vi "TC1014.vi"() -> ()   [LabVIEW 2019]
uses:
  SubVI/Typedef/TLibCANFD.ctl
panel:
  in  "启用4通道":bool
  in  "启用3通道":bool
  in  "启用2通道":bool
  in  "启用1通道":bool
  in  "选项卡控件":enum32{"CANFD1", "CANFD2", "CANFD3", "CANFD4"}(tab)
  in  "CH1  FD帧":u8(ring) items=["普通 CAN数据", "FD CAN数据"]
  in  "CH1显示报文类型":u16(ring)=1 items=["只读取接收的报文", "接收报文&发送报文"]
  in  "CH1终端电阻":u16(ring)=1 items=["Disable", "Enable"]
  in  "CH1物理通道":i32(ring) items=["CHN1", "CHN2", "CHN3", "CHN4", "CHN5", "CHN6", "CHN7", "CHN8", "CHN9", "CHN10", "CHN11", "CHN12", "CHN13", "CHN14", "CHN15", "CHN16", "CHN17", "CHN18", "CHN19", "CHN20", "CHN21", "CHN22", "CHN23", "CHN24", "CHN25", "CHN26", "CHN27", "CHN28", "CHN29", "CHN30", "CHN31", "CHN32"]
  in  "CH1应用程序逻辑通道":i32(ring) items=["CHN1", "CHN2", "CHN3", "CHN4", "CHN5", "CHN6", "CHN7", "CHN8", "CHN9", "CHN10", "CHN11", "CHN12", "CHN13", "CHN14", "CHN15", "CHN16", "CHN17", "CHN18", "CHN19", "CHN20", "CHN21", "CHN22", "CHN23", "CHN24", "CHN25", "CHN26", "CHN27", "CHN28", "CHN29", "CHN30", "CHN31", "CHN32"]
  in  "CH1仲裁域波特率":sgl=500.0 format="%#_g k"
  in  "CH1数据域波特率":sgl=2000.0 format="%#_g k"
  in  "CH1控制器类型":i32(ring)=1 items=["lfdtCAN", "lfdtISOFDCAN", "lfdtNonISOFDFDCAN"]
  in  "CH1控制器工作模式":i32(ring) items=["lfdmNormal", "lfdmACKOff", "lfdmRestricted"]
  in  "CH1发送":bool
  in  "CH1ID":i32 format="%x"
  in  "CH1帧格式":u8(ring) items=["标准帧", "扩展帧"]
  in  "CH1帧类型":u8(ring) items=["数据帧", "远程帧"]
  in  "CH1长度":u8
  in  "CH1SendData":u8[](array[numeric])=[0, 0, 0, 0, 0, 0, 0, 0, 0, 0, 0, 0, 0, 0, 0, 0, 0, 0, 0, 0, 0, 0, 0, 0, 0, 0, 0, 0, 0, 0, 0, 0, 0, 0, 0, 0, 0, 0, 0, 0, 0, 0, 0, 0, 0, 0, 0, 0, 0, 0, 0, 0, 0, 0, 0, 0, 0, 0, 0, 0, 0, 0, 0, 0, 0, 0, 0, 0, 0, 0, 0, 0, 0, 0, 0, 0] format="%x"
  in  "CH1Data":i32(listbox)=-1
  in  "CH2 FD帧 2":u8(ring) items=["普通 CAN数据", "FD CAN数据"]
  in  "CH2显示报文类型":u16(ring)=1 items=["Rx", "Rx&Tx"]
  in  "CH2终端电阻":u16(ring)=1 items=["Disable", "Enable"]
  in  "CH2物理通道":i32(ring)=1 items=["CHN1", "CHN2", "CHN3", "CHN4", "CHN5", "CHN6", "CHN7", "CHN8", "CHN9", "CHN10", "CHN11", "CHN12", "CHN13", "CHN14", "CHN15", "CHN16", "CHN17", "CHN18", "CHN19", "CHN20", "CHN21", "CHN22", "CHN23", "CHN24", "CHN25", "CHN26", "CHN27", "CHN28", "CHN29", "CHN30", "CHN31", "CHN32"]
  in  "CH2虚拟通道":i32(ring)=1 items=["CHN1", "CHN2", "CHN3", "CHN4", "CHN5", "CHN6", "CHN7", "CHN8", "CHN9", "CHN10", "CHN11", "CHN12", "CHN13", "CHN14", "CHN15", "CHN16", "CHN17", "CHN18", "CHN19", "CHN20", "CHN21", "CHN22", "CHN23", "CHN24", "CHN25", "CHN26", "CHN27", "CHN28", "CHN29", "CHN30", "CHN31", "CHN32"]
  in  "CH2仲裁域波特率":sgl=500.0 format="%#_g k"
  in  "CH2数据域波特率":sgl=2000.0 format="%#_g k"
  in  "CH2控制器类型":i32(ring) items=["lfdtCAN", "lfdtISOFDCAN", "lfdtNonISOFDFDCAN"]
  in  "CH2控制器工作模式":i32(ring) items=["lfdmNormal", "lfdmACKOff", "lfdmRestricted"]
  in  "CH2发送":bool
  in  "CH2ID":i32 format="%x"
  in  "CH2帧格式":u8(ring) items=["标准帧", "扩展帧"]
  in  "CH2帧类型":u8(ring) items=["数据帧", "远程帧"]
  in  "CH2长度":u8
  in  "CH2SendData":u8[](array[numeric])=[0, 0, 0, 0, 0, 0, 0, 0, 0, 0, 0, 0, 0, 0, 0, 0, 0, 0, 0, 0, 0, 0, 0, 0, 0, 0, 0, 0, 0, 0, 0, 0, 0, 0, 0, 0, 0, 0, 0, 0, 0, 0, 0, 0, 0, 0, 0, 0, 0, 0, 0, 0, 0, 0, 0, 0, 0, 0, 0, 0, 0, 0, 0, 0, 0, 0, 0, 0, 0, 0, 0, 0, 0, 0, 0, 0] format="%x"
  in  "CH2Data":i32(listbox)=-1
  in  "CH3 FD帧 3":u8(ring) items=["普通 CAN数据", "FD CAN数据"]
  in  "CH3显示报文类型":u16(ring)=1 items=["Rx", "Rx&Tx"]
  in  "CH3终端电阻":u16(ring)=1 items=["Disable", "Enable"]
  in  "CH3物理通道":i32(ring)=2 items=["CHN1", "CHN2", "CHN3", "CHN4", "CHN5", "CHN6", "CHN7", "CHN8", "CHN9", "CHN10", "CHN11", "CHN12", "CHN13", "CHN14", "CHN15", "CHN16", "CHN17", "CHN18", "CHN19", "CHN20", "CHN21", "CHN22", "CHN23", "CHN24", "CHN25", "CHN26", "CHN27", "CHN28", "CHN29", "CHN30", "CHN31", "CHN32"]
  in  "CH3虚拟通道":i32(ring)=2 items=["CHN1", "CHN2", "CHN3", "CHN4", "CHN5", "CHN6", "CHN7", "CHN8", "CHN9", "CHN10", "CHN11", "CHN12", "CHN13", "CHN14", "CHN15", "CHN16", "CHN17", "CHN18", "CHN19", "CHN20", "CHN21", "CHN22", "CHN23", "CHN24", "CHN25", "CHN26", "CHN27", "CHN28", "CHN29", "CHN30", "CHN31", "CHN32"]
  in  "CH3仲裁域波特率":sgl=500.0 format="%#_g k"
  in  "CH3数据域波特率":sgl=2000.0 format="%#_g k"
  in  "CH3控制器类型":i32(ring)=1 items=["lfdtCAN", "lfdtISOFDCAN", "lfdtNonISOFDFDCAN"]
  in  "CH3控制器工作模式":i32(ring) items=["lfdmNormal", "lfdmACKOff", "lfdmRestricted"]
  in  "CH3发送":bool
  in  "CH3ID":i32 format="%x"
  in  "CH3帧格式":u8(ring) items=["标准帧", "扩展帧"]
  in  "CH3帧类型":u8(ring) items=["数据帧", "远程帧"]
  in  "CH3长度":u8
  in  "CH3SendData":u8[](array[numeric])=[0, 0, 0, 0, 0, 0, 0, 0, 0, 0, 0, 0, 0, 0, 0, 0, 0, 0, 0, 0, 0, 0, 0, 0, 0, 0, 0, 0, 0, 0, 0, 0, 0, 0, 0, 0, 0, 0, 0, 0, 0, 0, 0, 0, 0, 0, 0, 0, 0, 0, 0, 0, 0, 0, 0, 0, 0, 0, 0, 0, 0, 0, 0, 0, 0, 0, 0, 0, 0, 0, 0, 0, 0, 0, 0, 0] format="%x"
  in  "CH3Data":i32(listbox)=-1
  in  "CH4 FD帧 3":u8(ring) items=["普通 CAN数据", "FD CAN数据"]
  in  "CH4显示报文类型":u16(ring)=1 items=["Rx", "Rx&Tx"]
  in  "CH4终端电阻":u16(ring)=1 items=["Disable", "Enable"]
  in  "CH4物理通道":i32(ring)=3 items=["CHN1", "CHN2", "CHN3", "CHN4", "CHN5", "CHN6", "CHN7", "CHN8", "CHN9", "CHN10", "CHN11", "CHN12", "CHN13", "CHN14", "CHN15", "CHN16", "CHN17", "CHN18", "CHN19", "CHN20", "CHN21", "CHN22", "CHN23", "CHN24", "CHN25", "CHN26", "CHN27", "CHN28", "CHN29", "CHN30", "CHN31", "CHN32"]
  in  "CH4虚拟通道":i32(ring)=3 items=["CHN1", "CHN2", "CHN3", "CHN4", "CHN5", "CHN6", "CHN7", "CHN8", "CHN9", "CHN10", "CHN11", "CHN12", "CHN13", "CHN14", "CHN15", "CHN16", "CHN17", "CHN18", "CHN19", "CHN20", "CHN21", "CHN22", "CHN23", "CHN24", "CHN25", "CHN26", "CHN27", "CHN28", "CHN29", "CHN30", "CHN31", "CHN32"]
  in  "CH4仲裁域波特率":sgl=500.0 format="%#_g k"
  in  "CH4数据域波特率":sgl=2000.0 format="%#_g k"
  in  "CH4控制器类型":i32(ring)=1 items=["lfdtCAN", "lfdtISOFDCAN", "lfdtNonISOFDFDCAN"]
  in  "CH4控制器工作模式":i32(ring) items=["lfdmNormal", "lfdmACKOff", "lfdmRestricted"]
  in  "CH4发送":bool
  in  "CH4ID":i32 format="%x"
  in  "CH4帧格式":u8(ring) items=["标准帧", "扩展帧"]
  in  "CH4帧类型":u8(ring) items=["数据帧", "远程帧"]
  in  "CH4长度":u8
  in  "CH4SendData":u8[](array[numeric])=[0, 0, 0, 0, 0, 0, 0, 0, 0, 0, 0, 0, 0, 0, 0, 0, 0, 0, 0, 0, 0, 0, 0, 0, 0, 0, 0, 0, 0, 0, 0, 0, 0, 0, 0, 0, 0, 0, 0, 0, 0, 0, 0, 0, 0, 0, 0, 0, 0, 0, 0, 0, 0, 0, 0, 0, 0, 0, 0, 0, 0, 0, 0, 0, 0, 0, 0, 0, 0, 0, 0, 0, 0, 0, 0, 0] format="%x"
  in  "CH4Data":i32(listbox)=-1
  out "通讯":bool
  in  "使用通道数量":u16(ring)=4 items=["1通道"=1, "2通道"=2, "3通道"=3, "4通道"=4, "5通道"=5]
  in  "硬件启闭":bool
  in  "退出程序":bool
  # "CAN DEMO_TC1014"
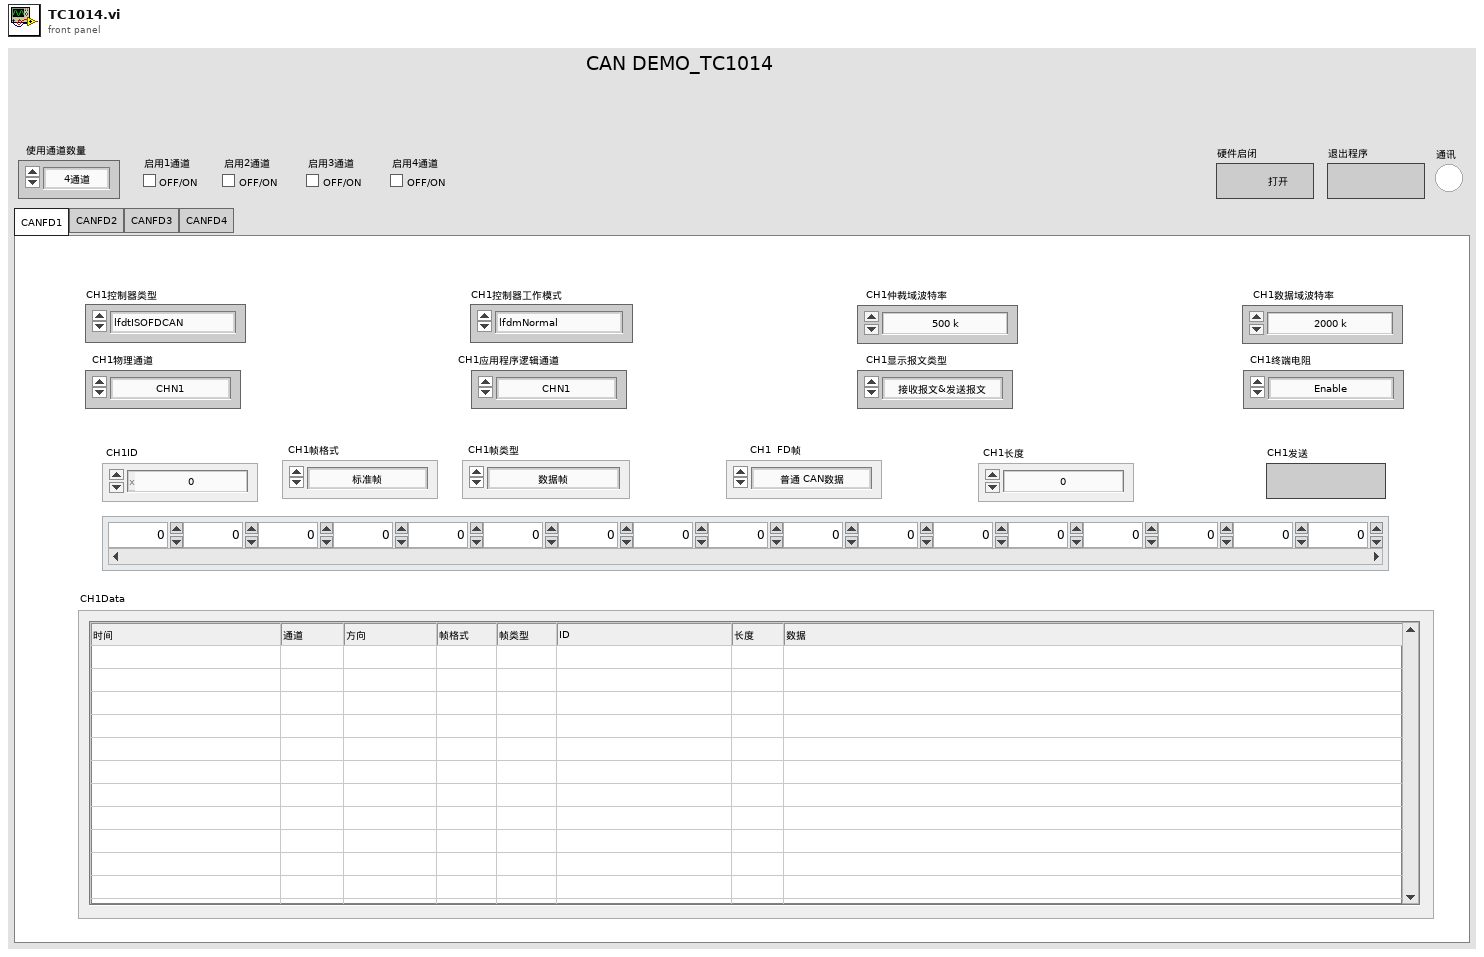
[diagram p1: front panel]
types:
  T1 = cluster{"AIdxchn":u8, "AId":i32, "AIsStd":u8, "AIsData":u8, "ADLC":u8, "簇":cluster{"初始化的数组[0]":u8, "初始化的数组[1]":u8, "初始化的数组[2]":u8, "初始化的数组[3]":u8, "初始化的数组[4]":u8, "初始化的数组[5]":u8, "初始化的数组[6]":u8, "初始化的数组[7]":u8, "初始化的数组[8]":u8, "初始化的数组[9]":u8, "初始化的数组[10]":u8, "初始化的数组[11]":u8, "初始化的数组[12]":u8, "初始化的数组[13]":u8, "初始化的数组[14]":u8, "初始化的数组[15]":u8, "初始化的数组[16]":u8, "初始化的数组[17]":u8, "初始化的数组[18]":u8, "初始化的数组[19]":u8, "初始化的数组[20]":u8, "初始化的数组[21]":u8, "初始化的数组[22]":u8, "初始化的数组[23]":u8, "初始化的数组[24]":u8, "初始化的数组[25]":u8, "初始化的数组[26]":u8, "初始化的数组[27]":u8, "初始化的数组[28]":u8, "初始化的数组[29]":u8, "初始化的数组[30]":u8, "初始化的数组[31]":u8, "初始化的数组[32]":u8, "初始化的数组[33]":u8, "初始化的数组[34]":u8, "初始化的数组[35]":u8, "初始化的数组[36]":u8, "初始化的数组[37]":u8, "初始化的数组[38]":u8, "初始化的数组[39]":u8, "初始化的数组[40]":u8, "初始化的数组[41]":u8, "初始化的数组[42]":u8, "初始化的数组[43]":u8, "初始化的数组[44]":u8, "初始化的数组[45]":u8, "初始化的数组[46]":u8, "初始化的数组[47]":u8, "初始化的数组[48]":u8, "初始化的数组[49]":u8, "初始化的数组[50]":u8, "初始化的数组[51]":u8, "初始化的数组[52]":u8, "初始化的数组[53]":u8, "初始化的数组[54]":u8, "初始化的数组[55]":u8, "初始化的数组[56]":u8, "初始化的数组[57]":u8, "初始化的数组[58]":u8, "初始化的数组[59]":u8, "初始化的数组[60]":u8, "初始化的数组[61]":u8, "初始化的数组[62]":u8, "初始化的数组[63]":u8, "初始化的数组[64] ":u8}}
  T2 = cluster{"FIdxChn":u8, "FProperties":u8, "FDLC":u8, "FReserved":u8, "FIdentifier":i32, "FTimeUS":u64, "簇":cluster{"初始化的数组[0]":u8, "初始化的数组[1]":u8, "初始化的数组[2]":u8, "初始化的数组[3]":u8, "初始化的数组[4]":u8, "初始化的数组[5]":u8, "初始化的数组[6]":u8, "初始化的数组[7]":u8, "初始化的数组[8]":u8, "初始化的数组[9]":u8, "初始化的数组[10]":u8, "初始化的数组[11]":u8, "初始化的数组[12]":u8, "初始化的数组[13]":u8, "初始化的数组[14]":u8, "初始化的数组[15]":u8, "初始化的数组[16]":u8, "初始化的数组[17]":u8, "初始化的数组[18]":u8, "初始化的数组[19]":u8, "初始化的数组[20]":u8, "初始化的数组[21]":u8, "初始化的数组[22]":u8, "初始化的数组[23]":u8, "初始化的数组[24]":u8, "初始化的数组[25]":u8, "初始化的数组[26]":u8, "初始化的数组[27]":u8, "初始化的数组[28]":u8, "初始化的数组[29]":u8, "初始化的数组[30]":u8, "初始化的数组[31]":u8, "初始化的数组[32]":u8, "初始化的数组[33]":u8, "初始化的数组[34]":u8, "初始化的数组[35]":u8, "初始化的数组[36]":u8, "初始化的数组[37]":u8, "初始化的数组[38]":u8, "初始化的数组[39]":u8, "初始化的数组[40]":u8, "初始化的数组[41]":u8, "初始化的数组[42]":u8, "初始化的数组[43]":u8, "初始化的数组[44]":u8, "初始化的数组[45]":u8, "初始化的数组[46]":u8, "初始化的数组[47]":u8, "初始化的数组[48]":u8, "初始化的数组[49]":u8, "初始化的数组[50]":u8, "初始化的数组[51]":u8, "初始化的数组[52]":u8, "初始化的数组[53]":u8, "初始化的数组[54]":u8, "初始化的数组[55]":u8, "初始化的数组[56]":u8, "初始化的数组[57]":u8, "初始化的数组[58]":u8, "初始化的数组[59]":u8, "初始化的数组[60]":u8, "初始化的数组[61]":u8, "初始化的数组[62]":u8, "初始化的数组[63]":u8}}[]
  T3 = cluster{"硬件类型":i32, "硬件子类型":i32, "AArbRateKbps":sgl, "AListenOnly":enum16{"Normal", "ListenOnly"}, "Int120Ohm":enum16{"Disable", "Enable"}, "EnableChannel":enum16{"Disable", "Enable"}, "AHwChannel":i32, "AAppChannel":i32, "ADataRateKbps":sgl, "AControllerType":i32, "AControllerMode":i32}
  T4 = typedef "TLibCANFD.ctl" = cluster{"AIdxchn":u8, "AId":i32, "AIsStd":u8, "AIsData":u8, "ADLC":u8, "AIsFD":enum16{"Classic CAN报文", "FD CAN报文"}, "FDatas":cluster{"初始化的数组[0]":u8, "初始化的数组[1]":u8, "初始化的数组[2]":u8, "初始化的数组[3]":u8, "初始化的数组[4]":u8, "初始化的数组[5]":u8, "初始化的数组[6]":u8, "初始化的数组[7]":u8, "初始化的数组[8]":u8, "初始化的数组[9]":u8, "初始化的数组[10]":u8, "初始化的数组[11]":u8, "初始化的数组[12]":u8, "初始化的数组[13]":u8, "初始化的数组[14]":u8, "初始化的数组[15]":u8, "初始化的数组[16]":u8, "初始化的数组[17]":u8, "初始化的数组[18]":u8, "初始化的数组[19]":u8, "初始化的数组[20]":u8, "初始化的数组[21]":u8, "初始化的数组[22]":u8, "初始化的数组[23]":u8, "初始化的数组[24]":u8, "初始化的数组[25]":u8, "初始化的数组[26]":u8, "初始化的数组[27]":u8, "初始化的数组[28]":u8, "初始化的数组[29]":u8, "初始化的数组[30]":u8, "初始化的数组[31]":u8, "初始化的数组[32]":u8, "初始化的数组[33]":u8, "初始化的数组[34]":u8, "初始化的数组[35]":u8, "初始化的数组[36]":u8, "初始化的数组[37]":u8, "初始化的数组[38]":u8, "初始化的数组[39]":u8, "初始化的数组[40]":u8, "初始化的数组[41]":u8, "初始化的数组[42]":u8, "初始化的数组[43]":u8, "初始化的数组[44]":u8, "初始化的数组[45]":u8, "初始化的数组[46]":u8, "初始化的数组[47]":u8, "初始化的数组[48]":u8, "初始化的数组[49]":u8, "初始化的数组[50]":u8, "初始化的数组[51]":u8, "初始化的数组[52]":u8, "初始化的数组[53]":u8, "初始化的数组[54]":u8, "初始化的数组[55]":u8, "初始化的数组[56]":u8, "初始化的数组[57]":u8, "初始化的数组[58]":u8, "初始化的数组[59]":u8, "初始化的数组[60]":u8, "初始化的数组[61]":u8, "初始化的数组[62]":u8, "初始化的数组[63]":u8, "初始化的数组[64] ":u8}}
  T5 = cluster{"CH1SendData[0]":u8, "CH1SendData[1]":u8, "CH1SendData[2]":u8, "CH1SendData[3]":u8, "CH1SendData[4]":u8, "CH1SendData[5]":u8, "CH1SendData[6]":u8, "CH1SendData[7]":u8, "CH1SendData[8]":u8, "CH1SendData[9]":u8, "CH1SendData[10]":u8, "CH1SendData[11]":u8, "CH1SendData[12]":u8, "CH1SendData[13]":u8, "CH1SendData[14]":u8, "CH1SendData[15]":u8, "CH1SendData[16]":u8, "CH1SendData[17]":u8, "CH1SendData[18]":u8, "CH1SendData[19]":u8, "CH1SendData[20]":u8, "CH1SendData[21]":u8, "CH1SendData[22]":u8, "CH1SendData[23]":u8, "CH1SendData[24]":u8, "CH1SendData[25]":u8, "CH1SendData[26]":u8, "CH1SendData[27]":u8, "CH1SendData[28]":u8, "CH1SendData[29]":u8, "CH1SendData[30]":u8, "CH1SendData[31]":u8, "CH1SendData[32]":u8, "CH1SendData[33]":u8, "CH1SendData[34]":u8, "CH1SendData[35]":u8, "CH1SendData[36]":u8, "CH1SendData[37]":u8, "CH1SendData[38]":u8, "CH1SendData[39]":u8, "CH1SendData[40]":u8, "CH1SendData[41]":u8, "CH1SendData[42]":u8, "CH1SendData[43]":u8, "CH1SendData[44]":u8, "CH1SendData[45]":u8, "CH1SendData[46]":u8, "CH1SendData[47]":u8, "CH1SendData[48]":u8, "CH1SendData[49]":u8, "CH1SendData[50]":u8, "CH1SendData[51]":u8, "CH1SendData[52]":u8, "CH1SendData[53]":u8, "CH1SendData[54]":u8, "CH1SendData[55]":u8, "CH1SendData[56]":u8, "CH1SendData[57]":u8, "CH1SendData[58]":u8, "CH1SendData[59]":u8, "CH1SendData[60]":u8, "CH1SendData[61]":u8, "CH1SendData[62]":u8, "CH1SendData[63]":u8, "CH1SendData[64]":u8}
  T6 = cluster{"FIdxChn":u8, "FProperties":u8, "FDLC":u8, "FReserved":u8, "FIdentifier":i32, "FTimeUS":u64, "FData":cluster{"Data0":u8, "Data1":u8, "Data2":u8, "Data3":u8, "Data4":u8, "Data5":u8, "Data6":u8, "Data7":u8}}[]
  T7 = cluster{"FIdxChn":u8, "FProperties":u8, "FDLC":u8, "FReserved":u8, "FIdentifier":i32, "FTimeUS":u64, "Fdata":cluster{"初始化的数组[0]":u8, "初始化的数组[1]":u8, "初始化的数组[2]":u8, "初始化的数组[3]":u8, "初始化的数组[4]":u8, "初始化的数组[5]":u8, "初始化的数组[6]":u8, "初始化的数组[7]":u8, "初始化的数组[8]":u8, "初始化的数组[9]":u8, "初始化的数组[10]":u8, "初始化的数组[11]":u8, "初始化的数组[12]":u8, "初始化的数组[13]":u8, "初始化的数组[14]":u8, "初始化的数组[15]":u8, "初始化的数组[16]":u8, "初始化的数组[17]":u8, "初始化的数组[18]":u8, "初始化的数组[19]":u8, "初始化的数组[20]":u8, "初始化的数组[21]":u8, "初始化的数组[22]":u8, "初始化的数组[23]":u8, "初始化的数组[24]":u8, "初始化的数组[25]":u8, "初始化的数组[26]":u8, "初始化的数组[27]":u8, "初始化的数组[28]":u8, "初始化的数组[29]":u8, "初始化的数组[30]":u8, "初始化的数组[31]":u8, "初始化的数组[32]":u8, "初始化的数组[33]":u8, "初始化的数组[34]":u8, "初始化的数组[35]":u8, "初始化的数组[36]":u8, "初始化的数组[37]":u8, "初始化的数组[38]":u8, "初始化的数组[39]":u8, "初始化的数组[40]":u8, "初始化的数组[41]":u8, "初始化的数组[42]":u8, "初始化的数组[43]":u8, "初始化的数组[44]":u8, "初始化的数组[45]":u8, "初始化的数组[46]":u8, "初始化的数组[47]":u8, "初始化的数组[48]":u8, "初始化的数组[49]":u8, "初始化的数组[50]":u8, "初始化的数组[51]":u8, "初始化的数组[52]":u8, "初始化的数组[53]":u8, "初始化的数组[54]":u8, "初始化的数组[55]":u8, "初始化的数组[56]":u8, "初始化的数组[57]":u8, "初始化的数组[58]":u8, "初始化的数组[59]":u8, "初始化的数组[60]":u8, "初始化的数组[61]":u8, "初始化的数组[62]":u8, "初始化的数组[63]":u8}}[]
  T8 = cluster{"CH2SendData[0]":u8, "CH2SendData[1]":u8, "CH2SendData[2]":u8, "CH2SendData[3]":u8, "CH2SendData[4]":u8, "CH2SendData[5]":u8, "CH2SendData[6]":u8, "CH2SendData[7]":u8, "CH2SendData[8]":u8, "CH2SendData[9]":u8, "CH2SendData[10]":u8, "CH2SendData[11]":u8, "CH2SendData[12]":u8, "CH2SendData[13]":u8, "CH2SendData[14]":u8, "CH2SendData[15]":u8, "CH2SendData[16]":u8, "CH2SendData[17]":u8, "CH2SendData[18]":u8, "CH2SendData[19]":u8, "CH2SendData[20]":u8, "CH2SendData[21]":u8, "CH2SendData[22]":u8, "CH2SendData[23]":u8, "CH2SendData[24]":u8, "CH2SendData[25]":u8, "CH2SendData[26]":u8, "CH2SendData[27]":u8, "CH2SendData[28]":u8, "CH2SendData[29]":u8, "CH2SendData[30]":u8, "CH2SendData[31]":u8, "CH2SendData[32]":u8, "CH2SendData[33]":u8, "CH2SendData[34]":u8, "CH2SendData[35]":u8, "CH2SendData[36]":u8, "CH2SendData[37]":u8, "CH2SendData[38]":u8, "CH2SendData[39]":u8, "CH2SendData[40]":u8, "CH2SendData[41]":u8, "CH2SendData[42]":u8, "CH2SendData[43]":u8, "CH2SendData[44]":u8, "CH2SendData[45]":u8, "CH2SendData[46]":u8, "CH2SendData[47]":u8, "CH2SendData[48]":u8, "CH2SendData[49]":u8, "CH2SendData[50]":u8, "CH2SendData[51]":u8, "CH2SendData[52]":u8, "CH2SendData[53]":u8, "CH2SendData[54]":u8, "CH2SendData[55]":u8, "CH2SendData[56]":u8, "CH2SendData[57]":u8, "CH2SendData[58]":u8, "CH2SendData[59]":u8, "CH2SendData[60]":u8, "CH2SendData[61]":u8, "CH2SendData[62]":u8, "CH2SendData[63]":u8, "CH2SendData[64]":u8}
  T9 = cluster{"CH3SendData[0]":u8, "CH3SendData[1]":u8, "CH3SendData[2]":u8, "CH3SendData[3]":u8, "CH3SendData[4]":u8, "CH3SendData[5]":u8, "CH3SendData[6]":u8, "CH3SendData[7]":u8, "CH3SendData[8]":u8, "CH3SendData[9]":u8, "CH3SendData[10]":u8, "CH3SendData[11]":u8, "CH3SendData[12]":u8, "CH3SendData[13]":u8, "CH3SendData[14]":u8, "CH3SendData[15]":u8, "CH3SendData[16]":u8, "CH3SendData[17]":u8, "CH3SendData[18]":u8, "CH3SendData[19]":u8, "CH3SendData[20]":u8, "CH3SendData[21]":u8, "CH3SendData[22]":u8, "CH3SendData[23]":u8, "CH3SendData[24]":u8, "CH3SendData[25]":u8, "CH3SendData[26]":u8, "CH3SendData[27]":u8, "CH3SendData[28]":u8, "CH3SendData[29]":u8, "CH3SendData[30]":u8, "CH3SendData[31]":u8, "CH3SendData[32]":u8, "CH3SendData[33]":u8, "CH3SendData[34]":u8, "CH3SendData[35]":u8, "CH3SendData[36]":u8, "CH3SendData[37]":u8, "CH3SendData[38]":u8, "CH3SendData[39]":u8, "CH3SendData[40]":u8, "CH3SendData[41]":u8, "CH3SendData[42]":u8, "CH3SendData[43]":u8, "CH3SendData[44]":u8, "CH3SendData[45]":u8, "CH3SendData[46]":u8, "CH3SendData[47]":u8, "CH3SendData[48]":u8, "CH3SendData[49]":u8, "CH3SendData[50]":u8, "CH3SendData[51]":u8, "CH3SendData[52]":u8, "CH3SendData[53]":u8, "CH3SendData[54]":u8, "CH3SendData[55]":u8, "CH3SendData[56]":u8, "CH3SendData[57]":u8, "CH3SendData[58]":u8, "CH3SendData[59]":u8, "CH3SendData[60]":u8, "CH3SendData[61]":u8, "CH3SendData[62]":u8, "CH3SendData[63]":u8, "CH3SendData[64]":u8}
  T10 = cluster{"CH4SendData[0]":u8, "CH4SendData[1]":u8, "CH4SendData[2]":u8, "CH4SendData[3]":u8, "CH4SendData[4]":u8, "CH4SendData[5]":u8, "CH4SendData[6]":u8, "CH4SendData[7]":u8, "CH4SendData[8]":u8, "CH4SendData[9]":u8, "CH4SendData[10]":u8, "CH4SendData[11]":u8, "CH4SendData[12]":u8, "CH4SendData[13]":u8, "CH4SendData[14]":u8, "CH4SendData[15]":u8, "CH4SendData[16]":u8, "CH4SendData[17]":u8, "CH4SendData[18]":u8, "CH4SendData[19]":u8, "CH4SendData[20]":u8, "CH4SendData[21]":u8, "CH4SendData[22]":u8, "CH4SendData[23]":u8, "CH4SendData[24]":u8, "CH4SendData[25]":u8, "CH4SendData[26]":u8, "CH4SendData[27]":u8, "CH4SendData[28]":u8, "CH4SendData[29]":u8, "CH4SendData[30]":u8, "CH4SendData[31]":u8, "CH4SendData[32]":u8, "CH4SendData[33]":u8, "CH4SendData[34]":u8, "CH4SendData[35]":u8, "CH4SendData[36]":u8, "CH4SendData[37]":u8, "CH4SendData[38]":u8, "CH4SendData[39]":u8, "CH4SendData[40]":u8, "CH4SendData[41]":u8, "CH4SendData[42]":u8, "CH4SendData[43]":u8, "CH4SendData[44]":u8, "CH4SendData[45]":u8, "CH4SendData[46]":u8, "CH4SendData[47]":u8, "CH4SendData[48]":u8, "CH4SendData[49]":u8, "CH4SendData[50]":u8, "CH4SendData[51]":u8, "CH4SendData[52]":u8, "CH4SendData[53]":u8, "CH4SendData[54]":u8, "CH4SendData[55]":u8, "CH4SendData[56]":u8, "CH4SendData[57]":u8, "CH4SendData[58]":u8, "CH4SendData[59]":u8, "CH4SendData[60]":u8, "CH4SendData[61]":u8, "CH4SendData[62]":u8, "CH4SendData[63]":u8, "CH4SendData[64]":u8}
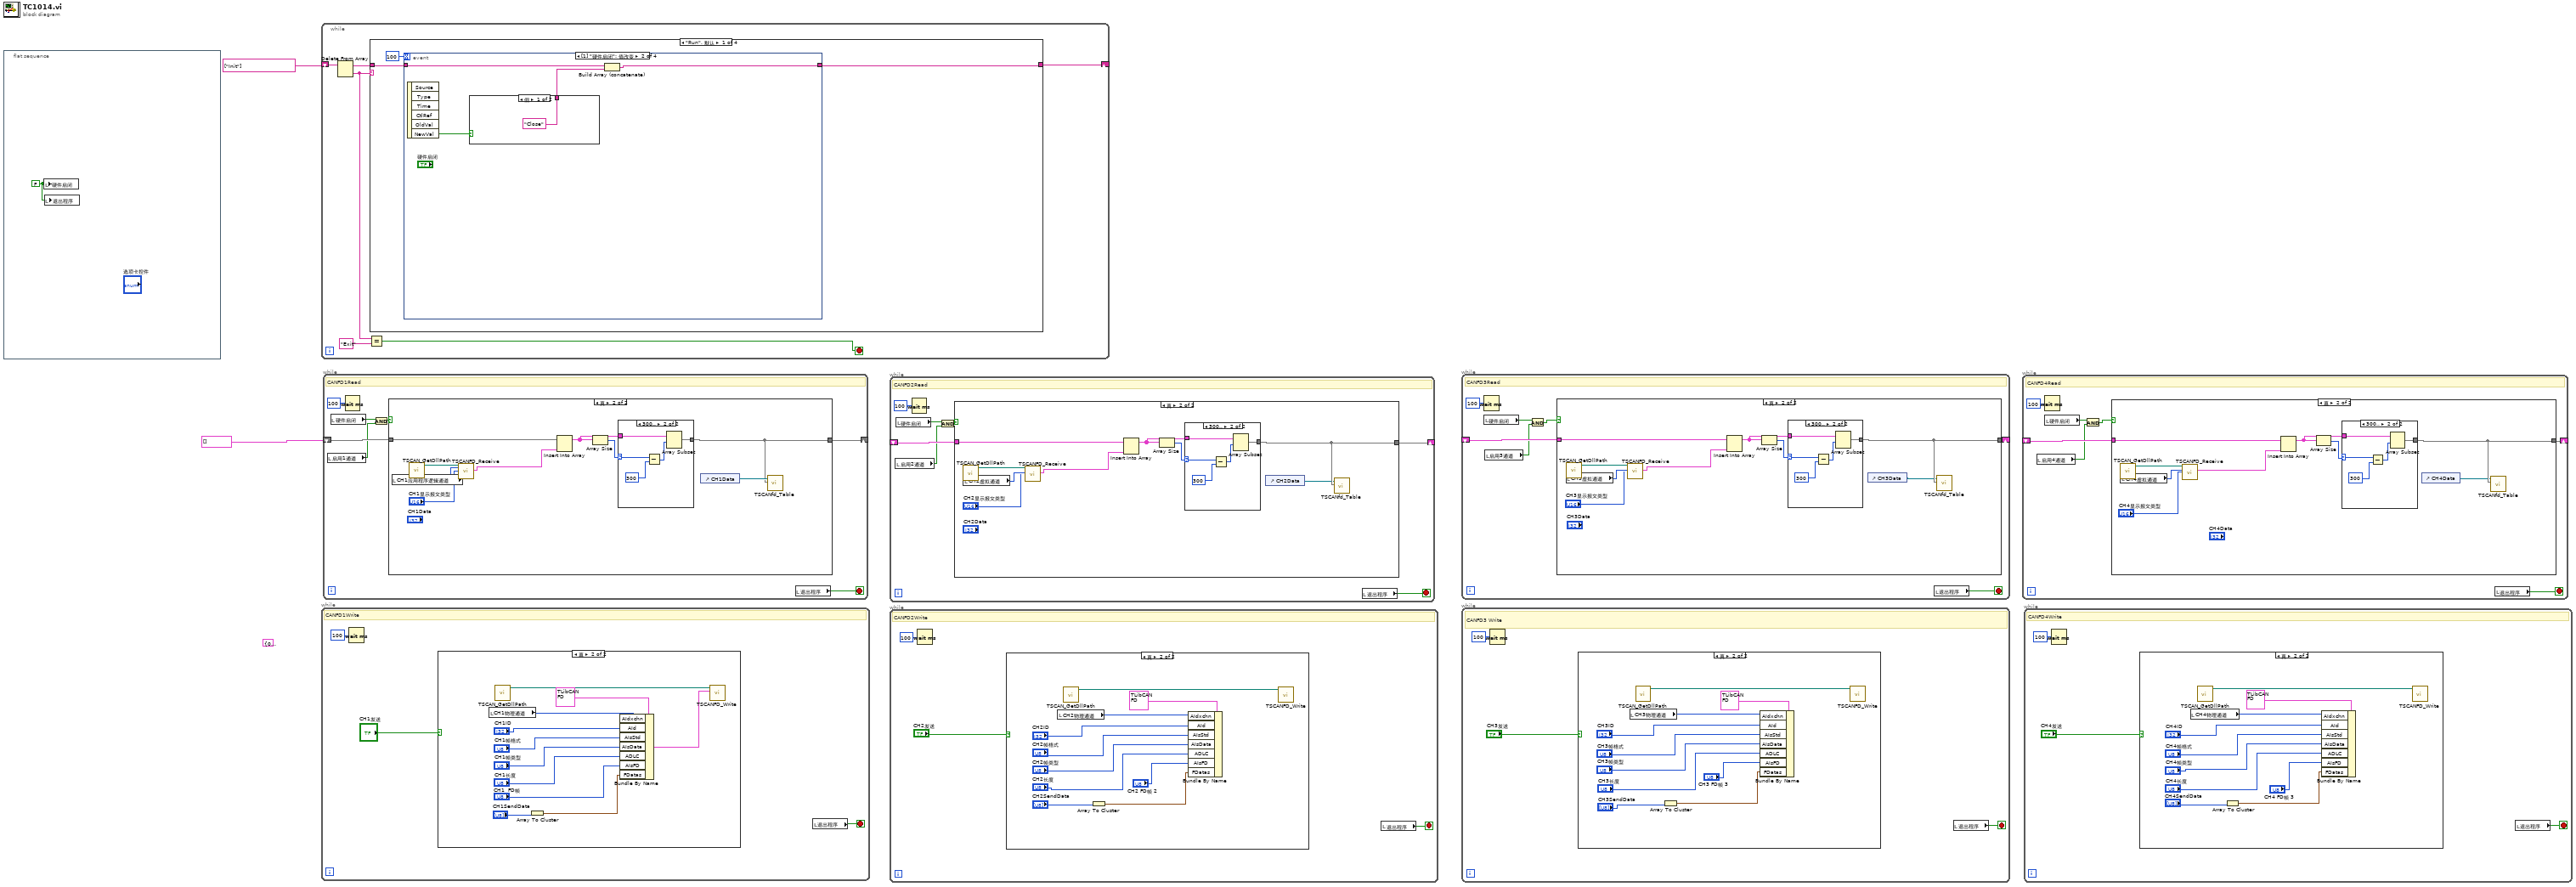
[diagram p0: block diagram]
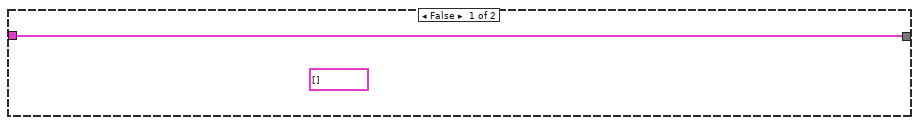
[diagram p3: hidden frame]
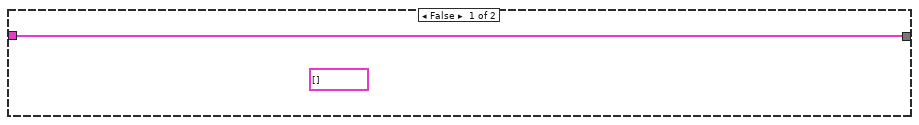
[diagram p6: hidden frame]
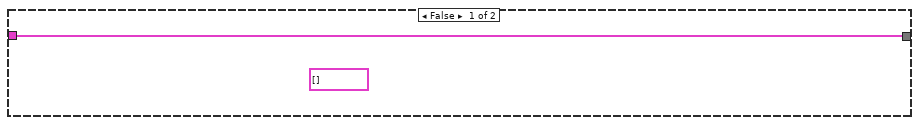
[diagram p9: hidden frame]
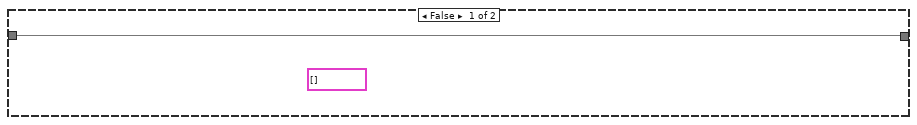
[diagram p12: hidden frame]
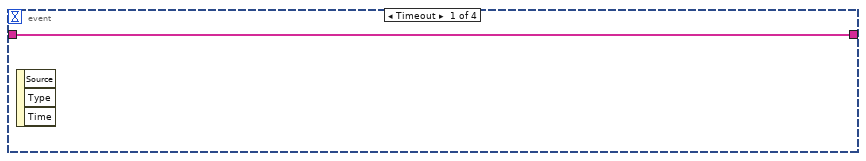
[diagram p14: hidden frame]
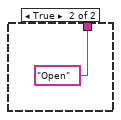
[diagram p15: hidden frame]
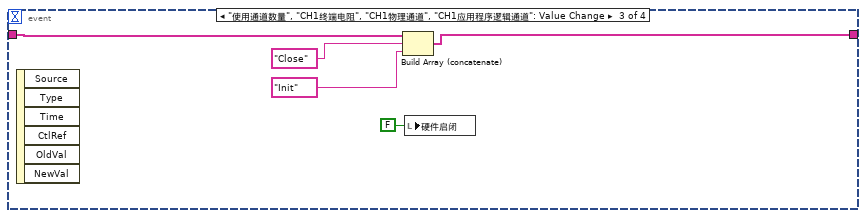
[diagram p16: hidden frame]
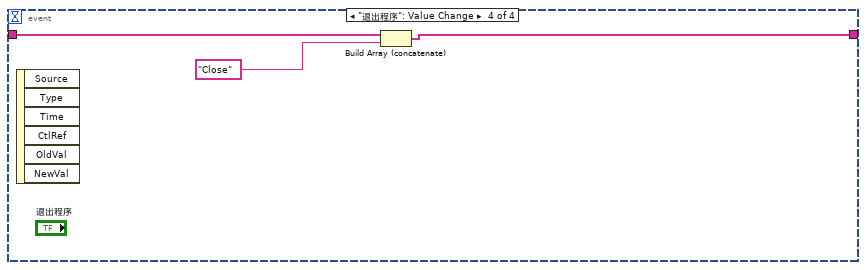
[diagram p17: hidden frame]
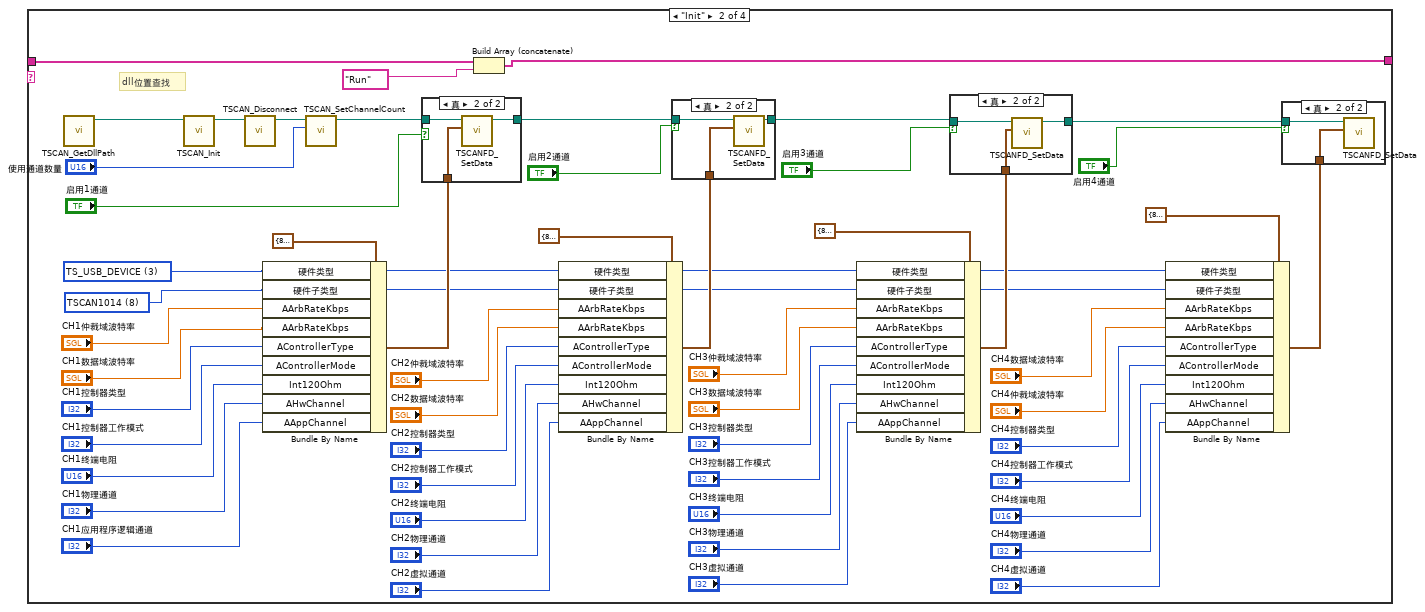
[diagram p18: hidden frame]
diagram:
  (unwired) T1 {"AIdxchn"=0, "AId"=0, "AIsStd"=0, "AIsData"=0, "ADLC"=0, "簇"={"初始化的数组[0]"=0, "初始化的数组[1]"=0, "初始化的数组[2]"=0, "初始化的数组[3]"=0, "初始化的数组[4]"=0, "初始化的数组[5]"=0, "初始化的数组[6]"=0, "初始化的数组[7]"=0, "初始化的数组[8]"=0, "初始化的数组[9]"=0, "初始化的数组[10]"=0, "初始化的数组[11]"=0, "初始化的数组[12]"=0, "初始化的数组[13]"=0, "初始化的数组[14]"=0, "初始化的数组[15]"=0, "初始化的数组[16]"=0, "初始化的数组[17]"=0, "初始化的数组[18]"=0, "初始化的数组[19]"=0, "初始化的数组[20]"=0, "初始化的数组[21]"=0, "初始化的数组[22]"=0, "初始化的数组[23]"=0, "初始化的数组[24]"=0, "初始化的数组[25]"=0, "初始化的数组[26]"=0, "初始化的数组[27]"=0, "初始化的数组[28]"=0, "初始化的数组[29]"=0, "初始化的数组[30]"=0, "初始化的数组[31]"=0, "初始化的数组[32]"=0, "初始化的数组[33]"=0, "初始化的数组[34]"=0, "初始化的数组[35]"=0, "初始化的数组[36]"=0, "初始化的数组[37]"=0, "初始化的数组[38]"=0, "初始化的数组[39]"=0, "初始化的数组[40]"=0, "初始化的数组[41]"=0, "初始化的数组[42]"=0, "初始化的数组[43]"=0, "初始化的数组[44]"=0, "初始化的数组[45]"=0, "初始化的数组[46]"=0, "初始化的数组[47]"=0, "初始化的数组[48]"=0, "初始化的数组[49]"=0, "初始化的数组[50]"=0, "初始化的数组[51]"=0, "初始化的数组[52]"=0, "初始化的数组[53]"=0, "初始化的数组[54]"=0, "初始化的数组[55]"=0, "初始化的数组[56]"=0, "初始化的数组[57]"=0, "初始化的数组[58]"=0, "初始化的数组[59]"=0, "初始化的数组[60]"=0, "初始化的数组[61]"=0, "初始化的数组[62]"=0, "初始化的数组[63]"=0, "初始化的数组[64] "=0}} ("TCAN 2")
  n1 = flat-sequence {
    frame #0 {
      w3 = FALSE ("硬件启闭")
      n2 = local write "硬件启闭"(w3) -> ()
      n3 = local write "退出程序"(w3) -> ()
    }
  }
  n4 = while {
    shift-right: [w7] -> _
    shift-left: string[] ["Init"] -> [w9]
    stop <- w4 stop-if-true
    n5 = Delete From Array(array=w9) -> (deleted portion=w6:string, array with subset deleted=w8:string[])  [unwired: 2 in]
    n6 = Equal?(x=w6, y="Exit") -> (x = y?=w4:bool)
    n7 = case shown="\"Run\", 默认" w6 {
      tunnel: w8 -> [w11 w75 w97 w104]
      tunnel: [w10 w74 w96 w105] -> w7
      frame "Run", Default {
        n8 = event shown="[1] \"硬件启闭\": 值改变" {
          selector: _ -> [_ _ _ _]
          dyn-events: _ -> [_ _ _ _]
          timeout: 100 -> [_ _ _ _]
          tunnel: w11 -> [w13 w17 w24 w26]
          tunnel: [w13 w16 w22 w25] -> w10
          event Timeout {
            n9 = event-data() -> ()  [unwired: 1 in, 3 out]
          }
          event "硬件启闭": Value Change {
            n10 = event-data() -> ("NewVal"=w15:bool)  [unwired: 1 in, 5 out]
            n11 = case shown="假" w15 {
              tunnel: ["Close" "Open"] -> w14
              frame False {
              }
              frame True {
              }
            }
            n12 = Build Array (concatenate)(w17, w14) -> (w16:string[])
          }
          event "使用通道数量", "CH1终端电阻", "CH1物理通道", "CH1应用程序逻辑通道": Value Change {
            n13 = event-data() -> ()  [unwired: 1 in, 6 out]
            n14 = Build Array (concatenate)(w24, "Close", "Init") -> (w22:string[])
            n15 = local write "硬件启闭"(FALSE ("硬件启闭")) -> ()
          }
          event "退出程序": Value Change {
            n16 = event-data() -> ()  [unwired: 1 in, 6 out]
            n17 = Build Array (concatenate)(w26, "Close") -> (w25:string[])
          }
        }
      }
      frame "Init" {
        w34 = 8 items=["BUS_UNKNOWN_TYPE", "TSCAN_PRO_4", "TSCAN_LITE_2", "TSCANMini", "TSLinMini", "TSCANFDmini", "TSCAN_LIN_IO_2", "TSCAN_LITE_2", "TSCAN1014", "TSCAN_FD_Mini_1"] ("硬件型号")
        w35 = 3 items=["BUS_UNKNOWN_TYPE", "TS_TCP_DEVICE", "XL_USB_DEVICE", "TS_USB_DEVICE", "PEAK_USB_DEVICE", "KVASER_USB_DEVICE", "ZLG_USB_DEVICE", "ICS_USB_DEVICE", "TS_TC1005_DEVICE"] ("硬件类型")
        # "dll位置查找"
        n18 = call "TSCAN_GetDllPath.vi"() -> ("DllPath"=w78:path)  [unwired: 11 in]
        n19 = call "TSCAN_Init.vi"("路径输入"=w78) -> ("路径输出"=w79:path)  [unwired: 8 in, 2 out]
        n20 = call "TSCAN_Disconnect.vi"("路径输入"=w79) -> ("路径输出"=w80:path)  [unwired: 9 in, 1 out]
        n21 = Bundle By Name(cluster=T3 {"硬件类型"=8, "硬件子类型"=0, "AArbRateKbps"=250.0, "AListenOnly"=enum."Normal", "Int120Ohm"=enum."Enable", "EnableChannel"=enum."Enable", "AHwChannel"=0, "AAppChannel"=0, "ADataRateKbps"=250.0, "AControllerType"=0, "AControllerMode"=0} ("CANFD配置"), "硬件类型"=w35, "硬件子类型"=w34, "AArbRateKbps"="CH1仲裁域波特率", "AArbRateKbps"="CH1数据域波特率", "AControllerType"="CH1控制器类型", "AControllerMode"="CH1控制器工作模式", "Int120Ohm"="CH1终端电阻", "AHwChannel"="CH1物理通道", "AAppChannel"="CH1应用程序逻辑通道") -> (w64:T3)
        n22 = call "TSCAN_SetChannelCount.vi"("Aount"="使用通道数量", "路径输入"=w80) -> ("路径输出"=w73:path)  [unwired: 7 in, 2 out]
        n23 = case shown="真" "启用1通道" {
          tunnel: w73 -> [w91 w94]
          tunnel: w64 -> [_ w93]
          tunnel: [w91 w92] -> w63
          frame False {
          }
          frame True {
            n24 = call "TSCANFD_SetData.vi"("CANFD配置"=w93, "路径输入"=w94) -> ("路径输出"=w92:path)  [unwired: 5 in, 4 out]
          }
        }
        n25 = Build Array (concatenate)(w75, "Run") -> (w74:string[])
        n26 = Bundle By Name(cluster=T3 {"硬件类型"=8, "硬件子类型"=0, "AArbRateKbps"=250.0, "AListenOnly"=enum."Normal", "Int120Ohm"=enum."Enable", "EnableChannel"=enum."Enable", "AHwChannel"=0, "AAppChannel"=0, "ADataRateKbps"=250.0, "AControllerType"=0, "AControllerMode"=0} ("CANFD配置"), "硬件类型"=w35, "硬件子类型"=w34, "AArbRateKbps"="CH2仲裁域波特率", "AArbRateKbps"="CH2数据域波特率", "AControllerType"="CH2控制器类型", "AControllerMode"="CH2控制器工作模式", "Int120Ohm"="CH2终端电阻", "AHwChannel"="CH2物理通道", "AAppChannel"="CH2虚拟通道") -> (w58:T3)
        n27 = case shown="真" "启用2通道" {
          tunnel: w58 -> [_ w90]
          tunnel: w63 -> [w87 w89]
          tunnel: [w87 w88] -> w50
          frame False {
          }
          frame True {
            n28 = call "TSCANFD_SetData.vi"("CANFD配置"=w90, "路径输入"=w89) -> ("路径输出"=w88:path)  [unwired: 5 in, 4 out]
          }
        }
        n29 = Bundle By Name(cluster=T3 {"硬件类型"=8, "硬件子类型"=0, "AArbRateKbps"=250.0, "AListenOnly"=enum."Normal", "Int120Ohm"=enum."Enable", "EnableChannel"=enum."Enable", "AHwChannel"=0, "AAppChannel"=0, "ADataRateKbps"=250.0, "AControllerType"=0, "AControllerMode"=0} ("CANFD配置"), "硬件类型"=w35, "硬件子类型"=w34, "AArbRateKbps"="CH3仲裁域波特率", "AArbRateKbps"="CH3数据域波特率", "AControllerType"="CH3控制器类型", "AControllerMode"="CH3控制器工作模式", "Int120Ohm"="CH3终端电阻", "AHwChannel"="CH3物理通道", "AAppChannel"="CH3虚拟通道") -> (w45:T3)
        n30 = case shown="真" "启用3通道" {
          tunnel: w50 -> [w83 w86]
          tunnel: [w83 w85] -> w49
          tunnel: w45 -> [_ w84]
          frame False {
          }
          frame True {
            n31 = call "TSCANFD_SetData.vi"("CANFD配置"=w84, "路径输入"=w86) -> ("路径输出"=w85:path)  [unwired: 5 in, 4 out]
          }
        }
        n32 = Bundle By Name(cluster=T3 {"硬件类型"=8, "硬件子类型"=0, "AArbRateKbps"=250.0, "AListenOnly"=enum."Normal", "Int120Ohm"=enum."Enable", "EnableChannel"=enum."Enable", "AHwChannel"=0, "AAppChannel"=0, "ADataRateKbps"=250.0, "AControllerType"=0, "AControllerMode"=0} ("CANFD配置"), "硬件类型"=w35, "硬件子类型"=w34, "AArbRateKbps"="CH4数据域波特率", "AArbRateKbps"="CH4仲裁域波特率", "AControllerType"="CH4控制器类型", "AControllerMode"="CH4控制器工作模式", "Int120Ohm"="CH4终端电阻", "AHwChannel"="CH4物理通道", "AAppChannel"="CH4虚拟通道") -> (w44:T3)
        n33 = case shown="真" "启用4通道" {
          tunnel: w44 -> [_ w82]
          tunnel: w49 -> [_ w81]
          frame False {
          }
          frame True {
            n34 = call "TSCANFD_SetData.vi"("CANFD配置"=w82, "路径输入"=w81) -> ()  [unwired: 5 in, 5 out]
          }
        }
      }
      frame "Open" {
        n35 = call "TSCAN_GetDllPath.vi"() -> ("DllPath"=w99:path)  [unwired: 11 in]
        n36 = call "TSCAN_Connect.vi"("路径输入"=w99) -> ("路径输出"=w100:path, "Connect_TSCAN_Successfully"=→"通讯":bool)  [unwired: 8 in, 1 out]
        n37 = Build Array (concatenate)(w97, "Run") -> (w96:string[])
        n38 = call "TSCAN_EnableReceive.vi"("路径输入"=w100) -> ()  [unwired: 9 in, 2 out]
      }
      frame "Close" {
        n39 = call "TSCAN_GetDllPath.vi"() -> ("DllPath"=w103:path)  [unwired: 11 in]
        n40 = local read "退出程序"() -> (w106:bool)
        n41 = local write "通讯"(FALSE ("通讯")) -> ()
        n42 = call "TSCAN_Close.vi"("路径输入"=w103) -> ("错误输出"=w102:errorcluster)  [unwired: 9 in, 1 out]
        n43 = case shown="假" w106 {
          tunnel: [w107 w111] -> w105
          tunnel: w104 -> [w108 w110]
          tunnel: w102 -> [_ _]
          frame False {
            n44 = Build Array (concatenate)(w108, "Run") -> (w107:string[])
          }
          frame True {
            n45 = Build Array (concatenate)(w110, "Exit") -> (w111:string[])
          }
        }
      }
    }
  }
  n46 = while {
    stop <- w115 stop-if-true
    # "CANFD1Write"
    n47 = Wait (ms)(milliseconds to wait=u32 100 ("等待时间（毫秒）")) -> ()  [unwired: 1 out]
    n48 = case shown="真" "CH1发送" {
      frame False {
      }
      frame True {
        n49 = local read "CH1物理通道"() -> (w121:i32)
        n50 = call "TSCAN_GetDllPath.vi"() -> ("DllPath"=w123:path)  [unwired: 11 in]
        n51 = Array To Cluster(array="CH1SendData") -> (cluster=w118:T5)
        n52 = Bundle By Name(cluster=T4 {"AIdxchn"=0, "AId"=0, "AIsStd"=0, "AIsData"=0, "ADLC"=0, "AIsFD"=enum."Classic CAN报文", "FDatas"={"初始化的数组[0]"=0, "初始化的数组[1]"=0, "初始化的数组[2]"=0, "初始化的数组[3]"=0, "初始化的数组[4]"=0, "初始化的数组[5]"=0, "初始化的数组[6]"=0, "初始化的数组[7]"=0, "初始化的数组[8]"=0, "初始化的数组[9]"=0, "初始化的数组[10]"=0, "初始化的数组[11]"=0, "初始化的数组[12]"=0, "初始化的数组[13]"=0, "初始化的数组[14]"=0, "初始化的数组[15]"=0, "初始化的数组[16]"=0, "初始化的数组[17]"=0, "初始化的数组[18]"=0, "初始化的数组[19]"=0, "初始化的数组[20]"=0, "初始化的数组[21]"=0, "初始化的数组[22]"=0, "初始化的数组[23]"=0, "初始化的数组[24]"=0, "初始化的数组[25]"=0, "初始化的数组[26]"=0, "初始化的数组[27]"=0, "初始化的数组[28]"=0, "初始化的数组[29]"=0, "初始化的数组[30]"=0, "初始化的数组[31]"=0, "初始化的数组[32]"=0, "初始化的数组[33]"=0, "初始化的数组[34]"=0, "初始化的数组[35]"=0, "初始化的数组[36]"=0, "初始化的数组[37]"=0, "初始化的数组[38]"=0, "初始化的数组[39]"=0, "初始化的数组[40]"=0, "初始化的数组[41]"=0, "初始化的数组[42]"=0, "初始化的数组[43]"=0, "初始化的数组[44]"=0, "初始化的数组[45]"=0, "初始化的数组[46]"=0, "初始化的数组[47]"=0, "初始化的数组[48]"=0, "初始化的数组[49]"=0, "初始化的数组[50]"=0, "初始化的数组[51]"=0, "初始化的数组[52]"=0, "初始化的数组[53]"=0, "初始化的数组[54]"=0, "初始化的数组[55]"=0, "初始化的数组[56]"=0, "初始化的数组[57]"=0, "初始化的数组[58]"=0, "初始化的数组[59]"=0, "初始化的数组[60]"=0, "初始化的数组[61]"=0, "初始化的数组[62]"=0, "初始化的数组[63]"=0, "初始化的数组[64] "=0}} ("TCANFD"), "AIdxchn"=w121, "AId"="CH1ID", "AIsStd"="CH1帧格式", "AIsData"="CH1帧类型", "ADLC"="CH1长度", "AIsFD"="CH1  FD帧", "FDatas"=w118) -> (w116:T4)
        n53 = call "TSCANFD_Write.vi"("TCANFD"=w116, "路径输入"=w123) -> ()  [unwired: 8 in, 2 out]
      }
    }
    n54 = local read "退出程序"() -> (w115:bool)
  }
  n55 = while {
    shift-right: [w130] -> _
    shift-left: T2 [] ("y") -> [w131]
    stop <- w133 stop-if-true
    # "CANFD1Read"
    n56 = local read "启用1通道"() -> (w128:bool)
    n57 = local read "硬件启闭"() -> (w129:bool)
    n58 = Wait (ms)(milliseconds to wait=u32 100 ("等待时间（毫秒）")) -> ()  [unwired: 1 out]
    n59 = And(x=w129, y=w128) -> (x .and. y?=w127:bool)
    n60 = case shown="真" w127 {
      tunnel: [w134 w136] -> w130
      tunnel: w131 -> [w134 w143]
      frame False {
        (unwired) T6 [] ("数组")
      }
      frame True {
        n61 = local read "CH1应用程序逻辑通道"() -> (w139:i32)
        n62 = call "TSCAN_GetDllPath.vi"() -> ("DllPath"=w140:path)  [unwired: 11 in]
        n63 = call "TSCANFD_Receive.vi"("显示报文类型"="CH1显示报文类型", "AAPPChannel"=w139, "路径输入"=w140) -> ("ACANMsgBuffer"=w135:T7)  [unwired: 5 in, 2 out]
        n64 = Insert Into Array(array=w143, new element=w135) -> (w141:T2)  [unwired: 1 in]
        n65 = Array Size(array=w141) -> (size(s)=w142:i32)
        n66 = case shown="300.." w142 {
          selector: w142 -> [_ w149]
          tunnel: [w144 w147] -> w136
          tunnel: w141 -> [w144 w145]
          frame 0, Default {
          }
          frame 300.. {
            n67 = Subtract(x=w149, y=300) -> (x-y=w146:i32)
            n68 = Array Subset(array=w145, index=w146) -> (w147:T2)  [unwired: 1 in]
          }
        }
        n69 = control-ref of="CH1Data"() -> (w137:refnum<vi>)
        n70 = call "TSCANfd_Table.vi"("y"=w136, "MCListbox引用句柄"=w137) -> ()  [unwired: 10 in]
      }
    }
    n71 = local read "退出程序"() -> (w133:bool)
  }
  n72 = while {
    shift-right: [w153] -> _
    shift-left: _ -> [w154]
    stop <- w156 stop-if-true
    # "CANFD2Read"
    n73 = local read "启用2通道"() -> (w150:bool)
    n74 = local read "硬件启闭"() -> (w152:bool)
    n75 = Wait (ms)(milliseconds to wait=u32 100 ("等待时间（毫秒）")) -> ()  [unwired: 1 out]
    n76 = And(x=w152, y=w150) -> (x .and. y?=w151:bool)
    n77 = case shown="真" w151 {
      tunnel: [w157 w162] -> w153
      tunnel: w154 -> [w157 w166]
      frame False {
        (unwired) T6 [] ("数组")
      }
      frame True {
        n78 = call "TSCAN_GetDllPath.vi"() -> ("DllPath"=w163:path)  [unwired: 11 in]
        n79 = local read "CH2虚拟通道"() -> (w160:i32)
        n80 = call "TSCANFD_Receive.vi"("显示报文类型"="CH2显示报文类型", "AAPPChannel"=w160, "路径输入"=w163) -> ("ACANMsgBuffer"=w158:T7)  [unwired: 5 in, 2 out]
        n81 = Insert Into Array(array=w166, new element=w158) -> (w164:T7)  [unwired: 1 in]
        n82 = Array Size(array=w164) -> (size(s)=w165:i32)
        n83 = case shown="300.." w165 {
          selector: w165 -> [_ w172]
          tunnel: [w167 w170] -> w162
          tunnel: w164 -> [w167 w168]
          frame 0, Default {
          }
          frame 300.. {
            n84 = Subtract(x=w172, y=300) -> (x-y=w169:i32)
            n85 = Array Subset(array=w168, index=w169) -> (w170:T7)  [unwired: 1 in]
          }
        }
        n86 = control-ref of="CH2Data"() -> (w161:refnum<vi>)
        n87 = call "TSCANfd_Table.vi"("y"=w162, "MCListbox引用句柄"=w161) -> ()  [unwired: 10 in]
      }
    }
    n88 = local read "退出程序"() -> (w156:bool)
  }
  n89 = while {
    stop <- w175 stop-if-true
    # "CANFD2Write"
    n90 = Wait (ms)(milliseconds to wait=u32 100 ("等待时间（毫秒）")) -> ()  [unwired: 1 out]
    n91 = case shown="真" "CH2发送" {
      frame False {
      }
      frame True {
        n92 = local read "CH2物理通道"() -> (w184:i32)
        n93 = call "TSCAN_GetDllPath.vi"() -> ("DllPath"=w185:path)  [unwired: 11 in]
        n94 = Array To Cluster(array="CH2SendData") -> (cluster=w177:T8)
        n95 = Bundle By Name(cluster=T4 {"AIdxchn"=0, "AId"=0, "AIsStd"=0, "AIsData"=0, "ADLC"=0, "AIsFD"=enum."Classic CAN报文", "FDatas"={"初始化的数组[0]"=0, "初始化的数组[1]"=0, "初始化的数组[2]"=0, "初始化的数组[3]"=0, "初始化的数组[4]"=0, "初始化的数组[5]"=0, "初始化的数组[6]"=0, "初始化的数组[7]"=0, "初始化的数组[8]"=0, "初始化的数组[9]"=0, "初始化的数组[10]"=0, "初始化的数组[11]"=0, "初始化的数组[12]"=0, "初始化的数组[13]"=0, "初始化的数组[14]"=0, "初始化的数组[15]"=0, "初始化的数组[16]"=0, "初始化的数组[17]"=0, "初始化的数组[18]"=0, "初始化的数组[19]"=0, "初始化的数组[20]"=0, "初始化的数组[21]"=0, "初始化的数组[22]"=0, "初始化的数组[23]"=0, "初始化的数组[24]"=0, "初始化的数组[25]"=0, "初始化的数组[26]"=0, "初始化的数组[27]"=0, "初始化的数组[28]"=0, "初始化的数组[29]"=0, "初始化的数组[30]"=0, "初始化的数组[31]"=0, "初始化的数组[32]"=0, "初始化的数组[33]"=0, "初始化的数组[34]"=0, "初始化的数组[35]"=0, "初始化的数组[36]"=0, "初始化的数组[37]"=0, "初始化的数组[38]"=0, "初始化的数组[39]"=0, "初始化的数组[40]"=0, "初始化的数组[41]"=0, "初始化的数组[42]"=0, "初始化的数组[43]"=0, "初始化的数组[44]"=0, "初始化的数组[45]"=0, "初始化的数组[46]"=0, "初始化的数组[47]"=0, "初始化的数组[48]"=0, "初始化的数组[49]"=0, "初始化的数组[50]"=0, "初始化的数组[51]"=0, "初始化的数组[52]"=0, "初始化的数组[53]"=0, "初始化的数组[54]"=0, "初始化的数组[55]"=0, "初始化的数组[56]"=0, "初始化的数组[57]"=0, "初始化的数组[58]"=0, "初始化的数组[59]"=0, "初始化的数组[60]"=0, "初始化的数组[61]"=0, "初始化的数组[62]"=0, "初始化的数组[63]"=0, "初始化的数组[64] "=0}} ("TCANFD"), "AIdxchn"=w184, "AId"="CH2ID", "AIsStd"="CH2帧格式", "AIsData"="CH2帧类型", "ADLC"="CH2长度", "AIsFD"="CH2 FD帧 2", "FDatas"=w177) -> ()  [unwired: 1 out]
        n96 = call "TSCANFD_Write.vi"("路径输入"=w185) -> ()  [unwired: 9 in, 2 out]
      }
    }
    n97 = local read "退出程序"() -> (w175:bool)
  }
  n98 = while {
    shift-right: [w189] -> _
    shift-left: _ -> [w190]
    stop <- w192 stop-if-true
    # "CANFD3Read"
    n99 = Wait (ms)(milliseconds to wait=u32 100 ("等待时间（毫秒）")) -> ()  [unwired: 1 out]
    n100 = local read "硬件启闭"() -> (w188:bool)
    n101 = local read "启用3通道"() -> (w187:bool)
    n102 = And(x=w188, y=w187) -> (x .and. y?=w186:bool)
    n103 = case shown="真" w186 {
      tunnel: [w193 w198] -> w189
      tunnel: w190 -> [w193 w202]
      frame False {
        (unwired) T6 [] ("数组")
      }
      frame True {
        n104 = call "TSCAN_GetDllPath.vi"() -> ("DllPath"=w199:path)  [unwired: 11 in]
        n105 = local read "CH3虚拟通道"() -> (w197:i32)
        n106 = call "TSCANFD_Receive.vi"("显示报文类型"="CH3显示报文类型", "AAPPChannel"=w197, "路径输入"=w199) -> ("ACANMsgBuffer"=w194:T7)  [unwired: 5 in, 2 out]
        n107 = Insert Into Array(array=w202, new element=w194) -> (w200:T7)  [unwired: 1 in]
        n108 = Array Size(array=w200) -> (size(s)=w201:i32)
        n109 = case shown="300.." w201 {
          selector: w201 -> [_ w208]
          tunnel: [w203 w206] -> w198
          tunnel: w200 -> [w203 w204]
          frame 0, Default {
          }
          frame 300.. {
            n110 = Subtract(x=w208, y=300) -> (x-y=w205:i32)
            n111 = Array Subset(array=w204, index=w205) -> (w206:T7)  [unwired: 1 in]
          }
        }
        n112 = control-ref of="CH3Data"() -> (w195:refnum<vi>)
        n113 = call "TSCANfd_Table.vi"("y"=w198, "MCListbox引用句柄"=w195) -> ()  [unwired: 10 in]
      }
    }
    n114 = local read "退出程序"() -> (w192:bool)
  }
  n115 = while {
    stop <- w211 stop-if-true
    # "CANFD3 Write"
    n116 = Wait (ms)(milliseconds to wait=u32 100 ("等待时间（毫秒）")) -> ()  [unwired: 1 out]
    n117 = case shown="真" "CH3发送" {
      frame False {
      }
      frame True {
        n118 = local read "CH3物理通道"() -> (w220:i32)
        n119 = call "TSCAN_GetDllPath.vi"() -> ("DllPath"=w221:path)  [unwired: 11 in]
        n120 = Array To Cluster(array="CH3SendData") -> (cluster=w213:T9)
        n121 = Bundle By Name(cluster=T4 {"AIdxchn"=0, "AId"=0, "AIsStd"=0, "AIsData"=0, "ADLC"=0, "AIsFD"=enum."Classic CAN报文", "FDatas"={"初始化的数组[0]"=0, "初始化的数组[1]"=0, "初始化的数组[2]"=0, "初始化的数组[3]"=0, "初始化的数组[4]"=0, "初始化的数组[5]"=0, "初始化的数组[6]"=0, "初始化的数组[7]"=0, "初始化的数组[8]"=0, "初始化的数组[9]"=0, "初始化的数组[10]"=0, "初始化的数组[11]"=0, "初始化的数组[12]"=0, "初始化的数组[13]"=0, "初始化的数组[14]"=0, "初始化的数组[15]"=0, "初始化的数组[16]"=0, "初始化的数组[17]"=0, "初始化的数组[18]"=0, "初始化的数组[19]"=0, "初始化的数组[20]"=0, "初始化的数组[21]"=0, "初始化的数组[22]"=0, "初始化的数组[23]"=0, "初始化的数组[24]"=0, "初始化的数组[25]"=0, "初始化的数组[26]"=0, "初始化的数组[27]"=0, "初始化的数组[28]"=0, "初始化的数组[29]"=0, "初始化的数组[30]"=0, "初始化的数组[31]"=0, "初始化的数组[32]"=0, "初始化的数组[33]"=0, "初始化的数组[34]"=0, "初始化的数组[35]"=0, "初始化的数组[36]"=0, "初始化的数组[37]"=0, "初始化的数组[38]"=0, "初始化的数组[39]"=0, "初始化的数组[40]"=0, "初始化的数组[41]"=0, "初始化的数组[42]"=0, "初始化的数组[43]"=0, "初始化的数组[44]"=0, "初始化的数组[45]"=0, "初始化的数组[46]"=0, "初始化的数组[47]"=0, "初始化的数组[48]"=0, "初始化的数组[49]"=0, "初始化的数组[50]"=0, "初始化的数组[51]"=0, "初始化的数组[52]"=0, "初始化的数组[53]"=0, "初始化的数组[54]"=0, "初始化的数组[55]"=0, "初始化的数组[56]"=0, "初始化的数组[57]"=0, "初始化的数组[58]"=0, "初始化的数组[59]"=0, "初始化的数组[60]"=0, "初始化的数组[61]"=0, "初始化的数组[62]"=0, "初始化的数组[63]"=0, "初始化的数组[64] "=0}} ("TCANFD"), "AIdxchn"=w220, "AId"="CH3ID", "AIsStd"="CH3帧格式", "AIsData"="CH3帧类型", "ADLC"="CH3长度", "AIsFD"="CH3 FD帧 3", "FDatas"=w213) -> ()  [unwired: 1 out]
        n122 = call "TSCANFD_Write.vi"("路径输入"=w221) -> ()  [unwired: 9 in, 2 out]
      }
    }
    n123 = local read "退出程序"() -> (w211:bool)
  }
  n124 = while {
    shift-right: [w225] -> _
    shift-left: _ -> [w226]
    stop <- w228 stop-if-true
    # "CANFD4Read"
    n125 = local read "启用4通道"() -> (w222:bool)
    n126 = Wait (ms)(milliseconds to wait=u32 100 ("等待时间（毫秒）")) -> ()  [unwired: 1 out]
    n127 = local read "硬件启闭"() -> (w224:bool)
    n128 = And(x=w224, y=w222) -> (x .and. y?=w223:bool)
    n129 = case shown="真" w223 {
      tunnel: [w229 w234] -> w225
      tunnel: w226 -> [w229 w238]
      frame False {
        (unwired) T6 [] ("数组")
      }
      frame True {
        n130 = call "TSCAN_GetDllPath.vi"() -> ("DllPath"=w235:path)  [unwired: 11 in]
        n131 = local read "CH4虚拟通道"() -> (w233:i32)
        n132 = call "TSCANFD_Receive.vi"("显示报文类型"="CH4显示报文类型", "AAPPChannel"=w233, "路径输入"=w235) -> ("ACANMsgBuffer"=w230:T7)  [unwired: 5 in, 2 out]
        n133 = Insert Into Array(array=w238, new element=w230) -> (w236:T7)  [unwired: 1 in]
        n134 = Array Size(array=w236) -> (size(s)=w237:i32)
        n135 = case shown="300.." w237 {
          selector: w237 -> [_ w244]
          tunnel: [w239 w242] -> w234
          tunnel: w236 -> [w239 w240]
          frame 0, Default {
          }
          frame 300.. {
            n136 = Subtract(x=w244, y=300) -> (x-y=w241:i32)
            n137 = Array Subset(array=w240, index=w241) -> (w242:T7)  [unwired: 1 in]
          }
        }
        n138 = control-ref of="CH4Data"() -> (w231:refnum<vi>)
        n139 = call "TSCANfd_Table.vi"("y"=w234, "MCListbox引用句柄"=w231) -> ()  [unwired: 10 in]
      }
    }
    n140 = local read "退出程序"() -> (w228:bool)
  }
  n141 = while {
    stop <- w247 stop-if-true
    # "CANFD4Write"
    n142 = Wait (ms)(milliseconds to wait=u32 100 ("等待时间（毫秒）")) -> ()  [unwired: 1 out]
    n143 = case shown="真" "CH4发送" {
      frame False {
      }
      frame True {
        n144 = local read "CH4物理通道"() -> (w256:i32)
        n145 = call "TSCAN_GetDllPath.vi"() -> ("DllPath"=w257:path)  [unwired: 11 in]
        n146 = Array To Cluster(array="CH4SendData") -> (cluster=w249:T10)
        n147 = Bundle By Name(cluster=T4 {"AIdxchn"=0, "AId"=0, "AIsStd"=0, "AIsData"=0, "ADLC"=0, "AIsFD"=enum."Classic CAN报文", "FDatas"={"初始化的数组[0]"=0, "初始化的数组[1]"=0, "初始化的数组[2]"=0, "初始化的数组[3]"=0, "初始化的数组[4]"=0, "初始化的数组[5]"=0, "初始化的数组[6]"=0, "初始化的数组[7]"=0, "初始化的数组[8]"=0, "初始化的数组[9]"=0, "初始化的数组[10]"=0, "初始化的数组[11]"=0, "初始化的数组[12]"=0, "初始化的数组[13]"=0, "初始化的数组[14]"=0, "初始化的数组[15]"=0, "初始化的数组[16]"=0, "初始化的数组[17]"=0, "初始化的数组[18]"=0, "初始化的数组[19]"=0, "初始化的数组[20]"=0, "初始化的数组[21]"=0, "初始化的数组[22]"=0, "初始化的数组[23]"=0, "初始化的数组[24]"=0, "初始化的数组[25]"=0, "初始化的数组[26]"=0, "初始化的数组[27]"=0, "初始化的数组[28]"=0, "初始化的数组[29]"=0, "初始化的数组[30]"=0, "初始化的数组[31]"=0, "初始化的数组[32]"=0, "初始化的数组[33]"=0, "初始化的数组[34]"=0, "初始化的数组[35]"=0, "初始化的数组[36]"=0, "初始化的数组[37]"=0, "初始化的数组[38]"=0, "初始化的数组[39]"=0, "初始化的数组[40]"=0, "初始化的数组[41]"=0, "初始化的数组[42]"=0, "初始化的数组[43]"=0, "初始化的数组[44]"=0, "初始化的数组[45]"=0, "初始化的数组[46]"=0, "初始化的数组[47]"=0, "初始化的数组[48]"=0, "初始化的数组[49]"=0, "初始化的数组[50]"=0, "初始化的数组[51]"=0, "初始化的数组[52]"=0, "初始化的数组[53]"=0, "初始化的数组[54]"=0, "初始化的数组[55]"=0, "初始化的数组[56]"=0, "初始化的数组[57]"=0, "初始化的数组[58]"=0, "初始化的数组[59]"=0, "初始化的数组[60]"=0, "初始化的数组[61]"=0, "初始化的数组[62]"=0, "初始化的数组[63]"=0, "初始化的数组[64] "=0}} ("TCANFD"), "AIdxchn"=w256, "AId"="CH4ID", "AIsStd"="CH4帧格式", "AIsData"="CH4帧类型", "ADLC"="CH4长度", "AIsFD"="CH4 FD帧 3", "FDatas"=w249) -> ()  [unwired: 1 out]
        n148 = call "TSCANFD_Write.vi"("路径输入"=w257) -> ()  [unwired: 9 in, 2 out]
      }
    }
    n149 = local read "退出程序"() -> (w247:bool)
  }
